vi "GetCurrentVarArrTag.vi"(0 "VarIndexArr":T1) -> (1 "CurrentArrayTag":string, 2 "IndexTagArr":u64[](array[numeric]), 3 "TopLevelItemName":string)   [LabVIEW 2016]
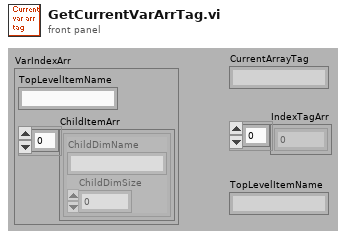
[diagram p1: front panel]
types:
  T1 = cluster{"TopLevelItemName":string, "ChildItemArr":cluster{"ChildDimName":string, "ChildDimSize":u64}[]}
  T2 = cluster{"ChildDimName":string, "ChildDimSize":u64}[]
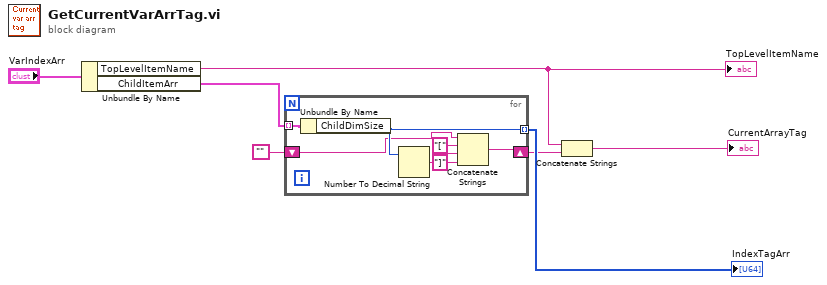
[diagram p0: block diagram]
diagram:
  n1 = Unbundle By Name("VarIndexArr") -> ("TopLevelItemName"=w6:string, "ChildItemArr"=w2:T2)
  "TopLevelItemName" <- w6
  n2 = for {
    tunnel: w2 -> [w14] mode=indexing
    tunnel: [w11] -> w7 mode=indexing
    shift-right: [w10] -> w4
    shift-left: "" -> [w9]
    n3 = Unbundle By Name(w14) -> ("ChildDimSize"=w11:u64)
    n4 = Number To Decimal String(number=w11) -> (decimal integer string=w8:string)  [unwired: 1 out]
    n5 = Concatenate Strings(w9, "[" ("字符串"), w8, "]" ("字符串")) -> (w10:string)
  }
  "IndexTagArr" <- w7
  n6 = Concatenate Strings(w6, w4) -> (→"CurrentArrayTag":string)
